vi "ConnectConfig.vi"(5 "service name":string, 6 "Decode type":T2=enum."Pupilometry", 7 "port":u16, 8 "error in (no error)":errorcluster, 9 "timeout ms (25000)":i32, 10 "byte order (0:big-endian, network order)":T1(ring), 11 "Smart_Eye_Pro_Driver in":refnum<class "SmartEyeProDriver.lvclass">) -> (0 "error out":errorcluster, 3 "Smart_Eye_Pro_Driver out":refnum<class "SmartEyeProDriver.lvclass">)   [LabVIEW 2020, in "SmartEyeProDriver.lvclass"]
uses:
  SmartEyeProDriver.lvclass
  Decode Class/Decode_Packet/Decode_type.ctl
  SmartEyeProDriver.lvclass/SmartEyeProDriver.ctl
  Decode Class/Decode_Packet/Decode_Packet.lvclass
  Decode Class/FrameInfo_class/FrameInfo.lvclass
  C:/Users/theod/Desktop/API - EyeT data streaming to IC/Smart Eye API/Source/Classes/Smart Eye Pro Drivers/Decode Class/Decode_Packet/Decode_Packet.lvclass
  Decode Class/Pupil_class/Pupil.lvclass
  Decode Class/Gaze_class/Gaze.lvclass
  Decode Class/AllInOne_class/AllInOne.lvclass
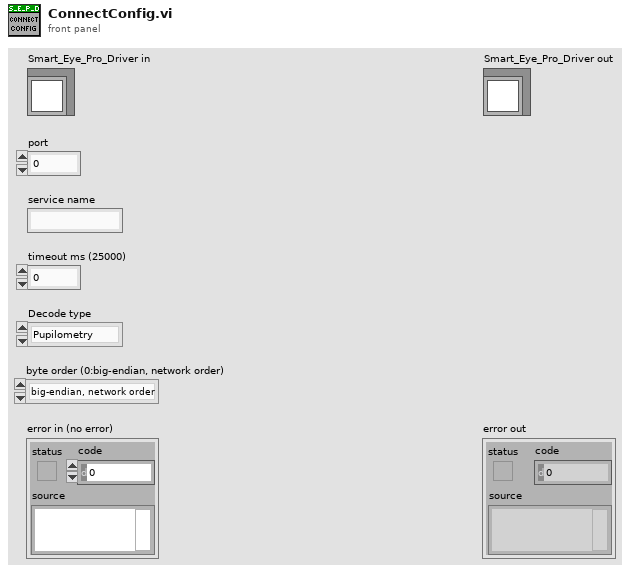
[diagram p1: front panel]
types:
  T1 = enum16{"big-endian, network order", "native, host order", "little-endian"}
  T2 = typedef "Decode_Packet.lvclass/Decode_type.ctl" = enum16{"Frame Information", "Raw Gaze", "Pupilometry", "All In One"}
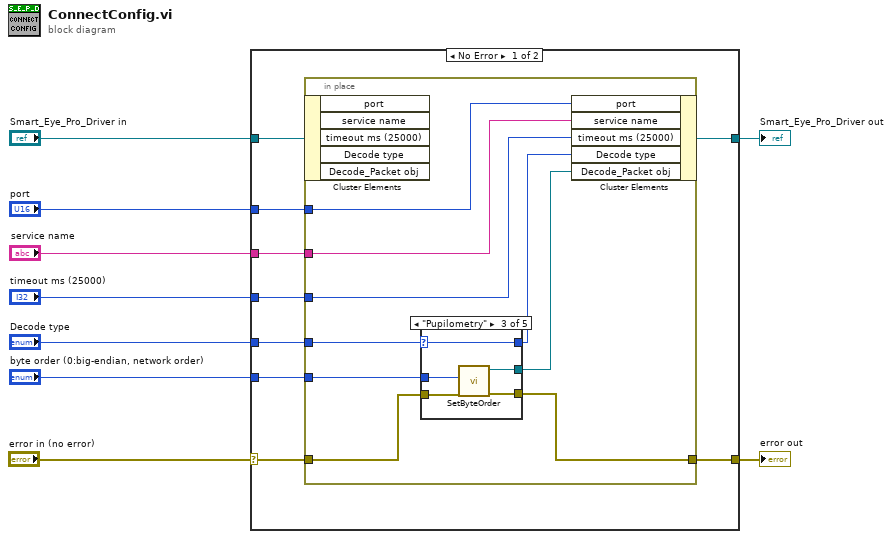
[diagram p0: block diagram]
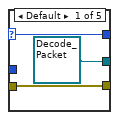
[diagram p2: hidden frame]
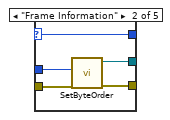
[diagram p3: hidden frame]
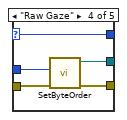
[diagram p4: hidden frame]
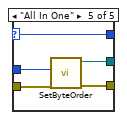
[diagram p5: hidden frame]
diagram:
  n1 = case shown="No Error" "error in (no error)" {
    selector: "error in (no error)" -> [w14 w51]
    tunnel: [w17 w52] -> w7
    tunnel: "Smart_Eye_Pro_Driver in" -> [w18 w52]
    tunnel: "port" -> [w11 _]
    tunnel: "service name" -> [w16 _]
    tunnel: "timeout ms (25000)" -> [w15 _]
    tunnel: [w13 w51] -> w3
    tunnel: "Decode type" -> [w12 _]
    tunnel: "byte order (0:big-endian, network order)" -> [w10 _]
    frame No Error {
      n2 = in-place {
        in-place-border: w16 -> [w27]
        in-place-border: w15 -> [w26]
        in-place-border: w14 -> [w20]
        in-place-border: [w19] -> w13
        in-place-border: w12 -> [w24]
        in-place-border: w11 -> [w25]
        in-place-border: w10 -> [w21]
        n3 = in-place-cluster #1(w18) -> ()  [unwired: 5 out]
        n4 = case shown="\"Pupilometry\"" w24 {
          selector: w24 -> [w30 w31 w36 w45 w50]
          tunnel: [w30 w31 w36 w45 w50] -> w23
          tunnel: [refnum<class "Decode_Packet.lvclass"> refnum ("Decode_Packet.lvclass") w34 w37 w44 w48] -> w22
          tunnel: w21 -> [_ w35 w40 w43 w49]
          tunnel: w20 -> [w29 w33 w39 w42 w47]
          tunnel: [w29 w32 w38 w41 w46] -> w19
          frame Default {
          }
          frame "Frame Information" {
            n5 = call "SetByteOrder.vi"("error in (no error)"=w33, "byte order (0:big-endian, network order)"=w35) -> ("error out"=w32:errorcluster, "Frame_Info out"=w34:refnum<class "FrameInfo.lvclass">)  [unwired: 8 in]
          }
          frame "Pupilometry" {
            n6 = call "SetByteOrder.vi"("error in (no error)"=w39, "byte order (0:big-endian, network order)"=w40) -> ("error out"=w38:errorcluster, "Pupil out"=w37:refnum<class "Pupil.lvclass">)  [unwired: 8 in]
          }
          frame "Raw Gaze" {
            n7 = call "SetByteOrder.vi"("error in (no error)"=w42, "byte order (0:big-endian, network order)"=w43) -> ("error out"=w41:errorcluster, "Gaze out"=w44:refnum<class "Gaze.lvclass">)  [unwired: 8 in]
          }
          frame "All In One" {
            n8 = call "SetByteOrder.vi"("error in (no error)"=w47, "byte order (0:big-endian, network order)"=w49) -> ("error out"=w46:errorcluster, "All_In_One out"=w48:refnum<class "AllInOne.lvclass">)  [unwired: 8 in]
          }
        }
        n9 = in-place-cluster #1("port"=w25, "service name"=w27, "timeout ms (25000)"=w26, "Decode type"=w23, "Decode_Packet obj"=w22) -> (w17:refnum<class "SmartEyeProDriver.lvclass">)
      }
    }
    frame Error {
    }
  }
  "error out" <- w3
  "Smart_Eye_Pro_Driver out" <- w7
